vi "retrieveConfiguration.vi"(8 "error in (no error)":errorcluster, 10 "dataName":string, 11 "WindowsTarget in":refnum<class "cRIOScanModeTarget.lvclass">) -> (0 "error out":errorcluster, 2 "dataValueFromFile":string, 3 "WindowsTarget out":refnum<class "cRIOScanModeTarget.lvclass">)   [LabVIEW 2012, in "cRIOScanModeTarget.lvclass"]
doc: "Retrieves the configuration data from the file associated with dataName."
uses:
  cRIOScanModeTarget.lvclass
  <vilib>/Utility/xml.llb/Read From XML File.vi
  <vilib>/Utility/xml.llb/Read From XML File(string).vi
  <userlib>/Common/ComponentModel/ComponentModelRT/ConfigurationFileReaderRT/ConfigurationFileReaderRT.lvclass
  <userlib>/Common/ComponentModel/ComponentModelDT/ConfigurationFileReaderDT/ConfigurationFileReaderDT.lvclass
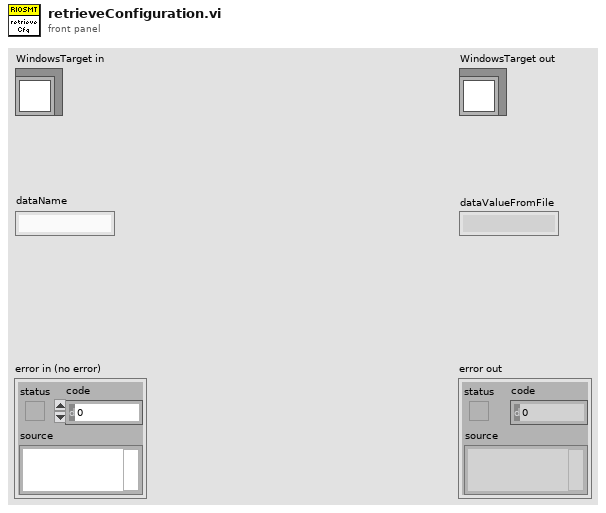
[diagram p1: front panel]
types:
  T1 = enum32{"invalid OS target", "Mac OS", "Windows 3.1", "Windows 95/NT", "Solaris 1", "Solaris 2", "HP-UX", "PowerMAX", "Linux", "Irix", "Rhapsody", "BeOS", "AIX", "OSF1", "VxWorks", "PharLap", "Carbon", "RTX", "Windows x64", "Linux x64"}
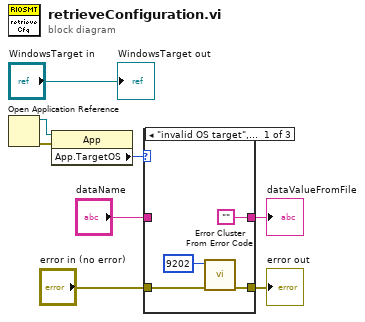
[diagram p0: block diagram]
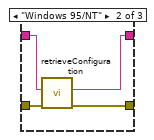
[diagram p2: hidden frame]
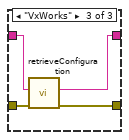
[diagram p3: hidden frame]
diagram:
  n1 = Open Application Reference() -> (0:w6:errorcluster, 3:w7:refnum<vi>)  [unwired: 4 in]
  n2 = property class="App"(reference=w7, error in=w6) -> ("App.TargetOS"=w5:T1)  [unwired: 2 out]
  n3 = case shown="\"invalid OS target\", Default" w5 {
    tunnel: "error in (no error)" -> [w11 w16 w20]
    tunnel: [w10 w15 w19] -> w3
    tunnel: "dataName" -> [_ w14 w18]
    tunnel: ["" w13 w17] -> w1
    frame "invalid OS target", Default {
      n4 = call <vilib>:"Error Cluster From Error Code.vi"("error in (no error)"=w11, "error code (0)"=9202) -> ("error out"=w10:errorcluster)  [unwired: 7 in]
    }
    frame "Windows 95/NT" {
      n5 = call <userlib>:"retrieveConfiguration.vi"("error in (no error)"=w16, "dataName"=w14) -> ("error out"=w15:errorcluster, "dataValueFromFile"=w13:string)  [unwired: 7 in, 1 out]
    }
    frame "VxWorks" {
      n6 = call <userlib>:"retrieveConfiguration.vi"("error in (no error)"=w20, "dataName"=w18) -> ("error out"=w19:errorcluster, "dataValueFromFile"=w17:string)  [unwired: 7 in, 1 out]
    }
  }
  "error out" <- w3
  "dataValueFromFile" <- w1
  "WindowsTarget out" <- "WindowsTarget in"
